vi "subKeepActiveTargetsOnly.vi"(8 "error in (no error)":errorcluster, 11 "SolutionBuilder in":refnum<class "SolutionBuilder.lvclass">) -> (0 "error out":errorcluster, 3 "SolutionBuilder out":refnum<class "SolutionBuilder.lvclass">)   [LabVIEW 2019, in "SolutionBuilder.lvlib" / "SolutionBuilder.lvclass"]
uses:
  SolutionBuilder.lvclass
  ProjectItem/ProjectItem.lvclass
  <vilib>/Utility/miscctls.llb/LVMapReplaceAction.ctl
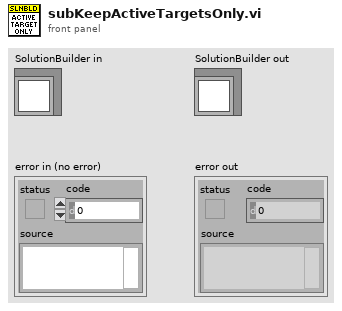
[diagram p1: front panel]
types:
  T1 = typedef "LVMapReplaceAction.ctl" = enum32{"Modify Entry only if found", "Add or Modify Entry", "Delete Entry"}
  T2 = typedef "SolutionBuilder.lvlib/SolutionBuilder.lvclass/ProjectItemMap.ctl" = map{path, refnum<class "ProjectItem.lvclass">[]}
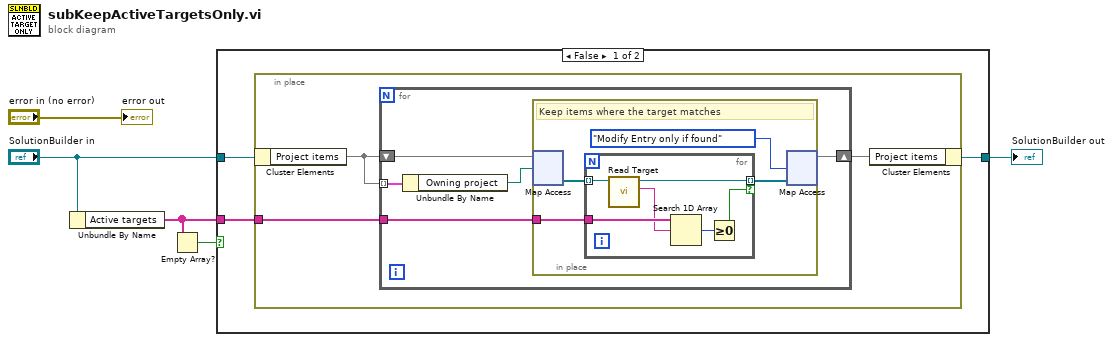
[diagram p0: block diagram]
diagram:
  n1 = Unbundle By Name("SolutionBuilder in") -> ("Active targets"=w3:string[])
  n2 = Empty Array?(array=w3) -> (empty?=w1:bool)
  n3 = case shown="False" w1 {
    tunnel: "SolutionBuilder in" -> [w8 w27]
    tunnel: w3 -> [w7 _]
    tunnel: [w6 w27] -> w2
    frame False {
      n4 = in-place {
        in-place-border: w7 -> [w10]
        n5 = in-place-cluster #1(w8) -> ("Project items"=w11:T2)
        n6 = for {
          tunnel: w11 -> [w16] mode=indexing
          shift-right: [w12] -> w9
          shift-left: w11 -> [w15]
          tunnel: w10 -> [w13]
          n7 = Unbundle By Name(w16) -> ("Owning project"=w14:path)
          n8 = in-place {
            in-place-border: w13 -> [w19]
            # "Keep items where the target matches"
            n9 = in-place-map #2(w15, w14) -> (w20:refnum<class "ProjectItem.lvclass">[])  [unwired: 1 in, 1 out]
            n10 = for {
              tunnel: w20 -> [w26] mode=indexing
              tunnel: w19 -> [w25]
              tunnel: [w22] -> w18 mode=indexing if=w21
              n11 = call "Read Target.vi"("ProjectItem in"=w26) -> ("Target"=w24:string, "ProjectItem out"=w22:refnum<class "ProjectItem.lvclass">)  [unwired: 9 in]
              n12 = Search 1D Array(1D array=w25, element=w24) -> (index of element=w23:i32)  [unwired: 1 in]
              n13 = Greater Or Equal To 0?(x=w23) -> (x >= 0?=w21:bool)
            }
            n14 = in-place-map #2(w18, LVMapReplaceAction."Modify Entry only if found" ("action")) -> (w12:T2)  [unwired: 2 out]
          }
        }
        n15 = in-place-cluster #1("Project items"=w9) -> (w6:refnum<class "SolutionBuilder.lvclass">)
      }
    }
    frame True {
    }
  }
  "SolutionBuilder out" <- w2
  "error out" <- "error in (no error)"
